vi "Unitary_Test_Open.vi"() -> (0 "Test_passed":bool)   [LabVIEW 2014]
panel:
  in  "expected results":T1(array[cluster])
  out "Results":T1(array[cluster])
  out "Test_OK":bool[](array[boolean])
  out "hidden":errorcluster
  in  "Array of imputs":string[](array[string])=["TestOK"]
  # "Test basic methods with some testing plant"
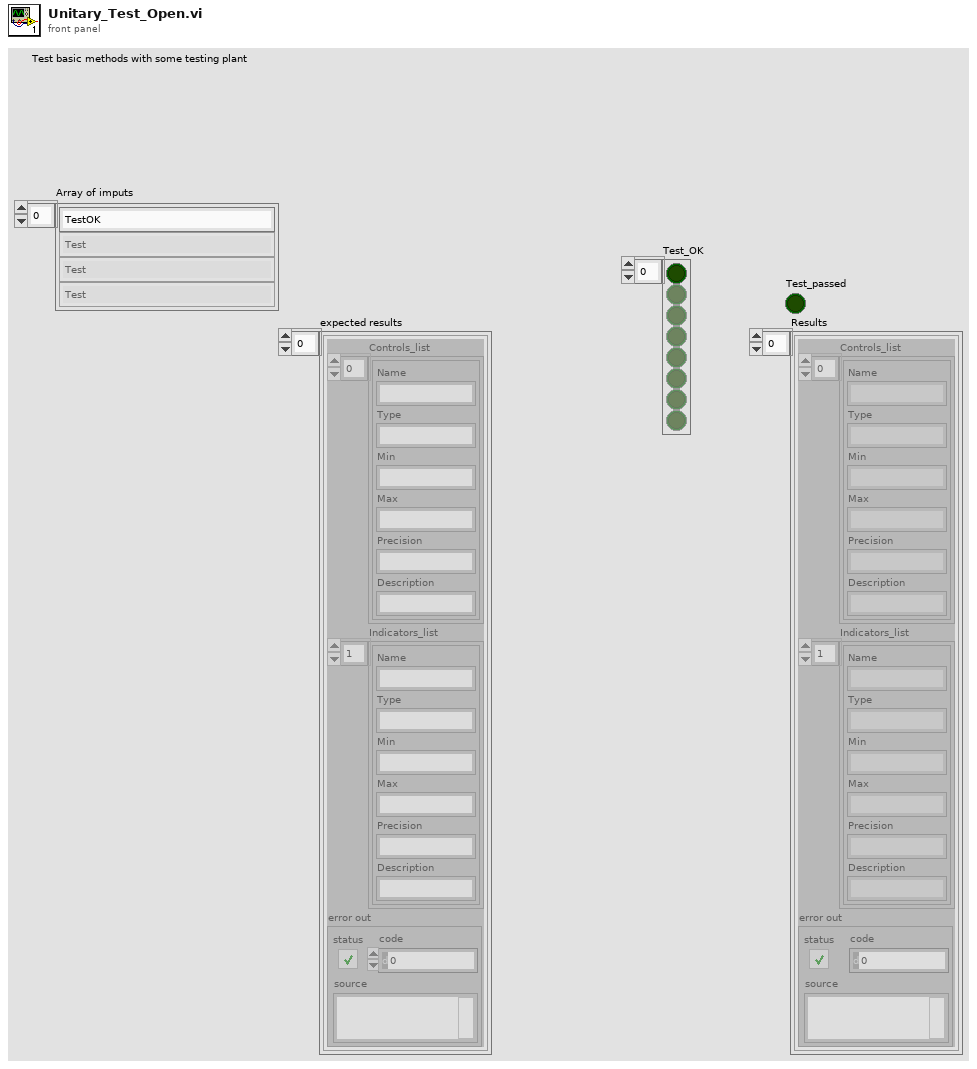
[diagram p1: front panel]
types:
  T1 = cluster{"Controls_list":cluster{"Name":string, "Type":string, "Min":string, "Max":string, "Precision":string, "Description":string}[], "Indicators_list":cluster{"Name":string, "Type":string, "Min":string, "Max":string, "Precision":string, "Description":string}[], "error out":errorcluster}[]
  T2 = cluster{"Name":string, "Type":string, "Min":string, "Max":string, "Precision":string, "Description":string}[]
  T3 = cluster{"Controls_list":cluster{"Name":string, "Type":string, "Min":string, "Max":string, "Precision":string, "Description":string}[], "Indicators_list":cluster{"Name":string, "Type":string, "Min":string, "Max":string, "Precision":string, "Description":string}[], "error out":errorcluster}
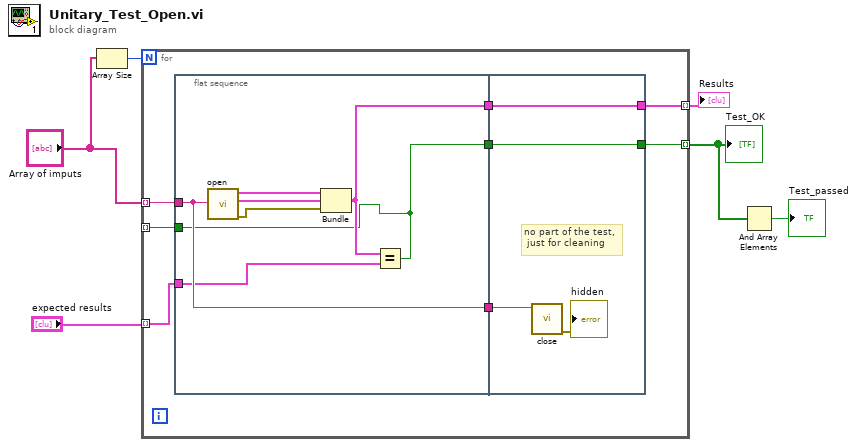
[diagram p0: block diagram]
diagram:
  n1 = Array Size(array="Array of imputs") -> (size(s)=w6:i32)
  n2 = for {
    N: w6 -> [_]
    tunnel: "Array of imputs" -> [w14] mode=indexing
    tunnel: [w12] -> w4 mode=indexing
    tunnel: [w10] -> w2 mode=indexing
    tunnel: "expected results" -> [w8] mode=indexing
    tunnel: [w7] -> _ mode=indexing
    n3 = flat-sequence {
      tunnel: w14 -> [w21]
      tunnel: [w21] -> w13
      tunnel: w8 -> [w17]
      tunnel: [w15] -> w11
      tunnel: [w16] -> w9
      tunnel: [w15] -> w7
      tunnel: w13 -> [w25]
      tunnel: [w23] -> w12
      tunnel: w11 -> [w23]
      tunnel: [w22] -> w10
      tunnel: w9 -> [w22]
      frame #0 {
        n4 = call "open.vi"("Experience ID"=w21) -> ("error out"=w18:errorcluster, "Indicators_list"=w19:T2, "Controls_list"=w20:T2)  [unwired: 8 in]
        n5 = Bundle("Controls_list"=w20, "Indicators_list"=w19, "error out"=w18) -> (w16:T3)  [unwired: 1 in]
        n6 = Equal?(x=w16, y=w17) -> (x = y?=w15:bool)
      }
      frame #1 {
        # "no part of the test,\n just for cleaning"
        n7 = call "close.vi"("Experience ID"=w25) -> ("error out"=→"hidden":errorcluster)  [unwired: 10 in]
      }
    }
  }
  "Test_OK" <- w4
  "Results" <- w2
  n8 = And Array Elements(Boolean array=w4) -> (logical AND=→"Test_passed":bool)
